vi "클라우드_날씨예보서비스.vi"() -> ()   [LabVIEW 2023]
uses:
  <vilib>/xml/Load XML String.vi
  <vilib>/xml/Close Reference(Node).vi
  System.Windows.Forms
  <vilib>/httpClient/LabVIEWHTTPClient.lvlib
  <vilib>/ni/Simple XML/Simple XML.lvlib
  <vilib>/xml/NI_XML.lvlib
  <resource>/objmgr/DOMUserDefRef.rc
panel:
  in  "격자 Y":string
  in  "격자 X":string
  out "초단기예보":T1(array[cluster])
  out "array":cluster{"이름":string, "node text":string}[][](array[cluster])
  out "Pretty XML String":string
  out "body":string
  out "header":string
  in  "경도":string
  in  "위도":string
  in  "새로고침":bool
  in  "정지 버튼":bool
  in  "웹 브라우저":refnum<k24>(container)
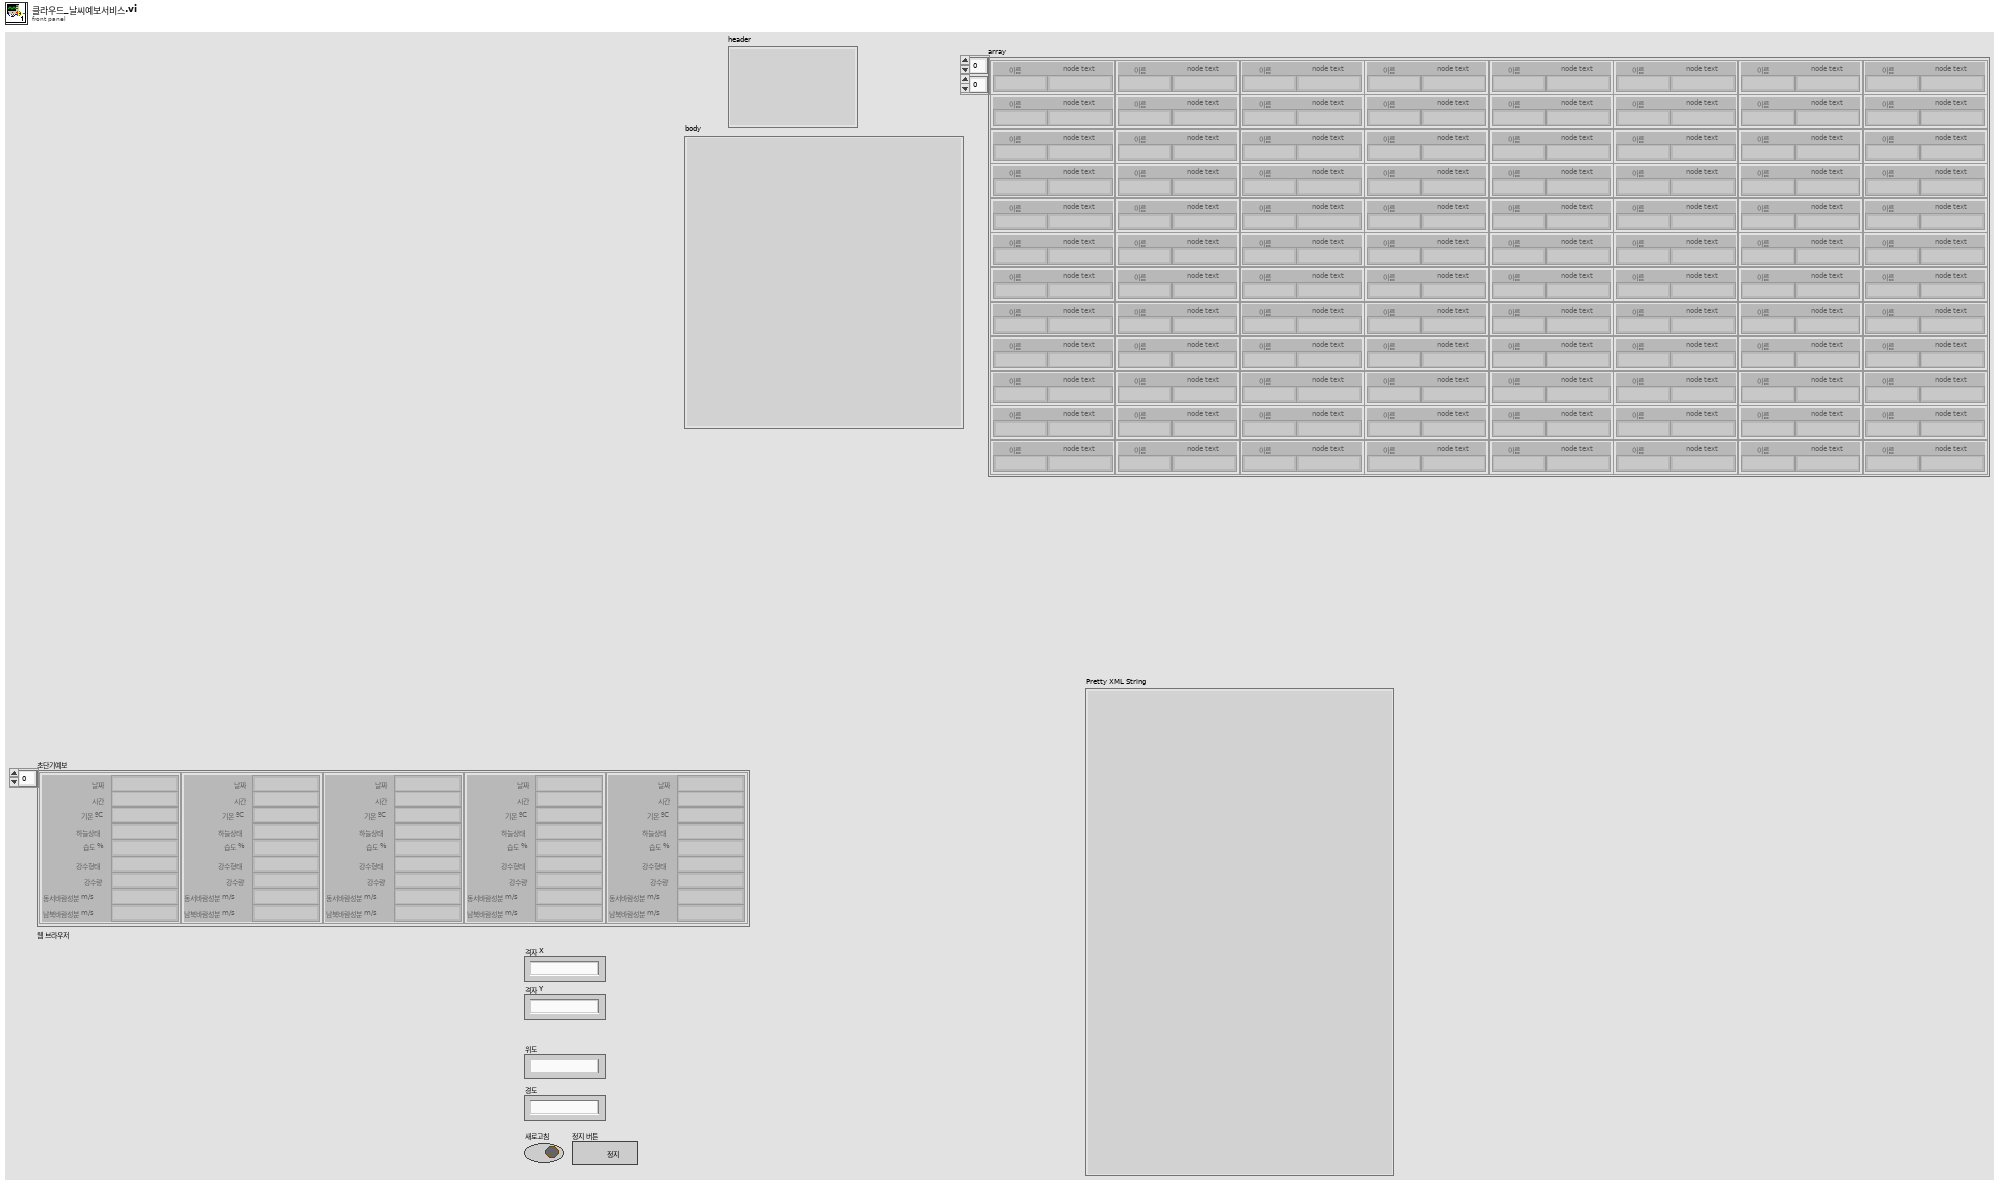
[diagram p1: front panel]
types:
  T1 = cluster{"날짜":string, "시간":string, "기온 ºC":string, "하늘상태":string, "습도 %":string, "강수형태":string, "강수량":string, "동서바람성분 m/s":string, "남북바람성분 m/s":string}[]
  T2 = cluster{"node text":string, "node text":string, "node text":string, string, "node text":string, string, string, "node text":string, "node text":string}
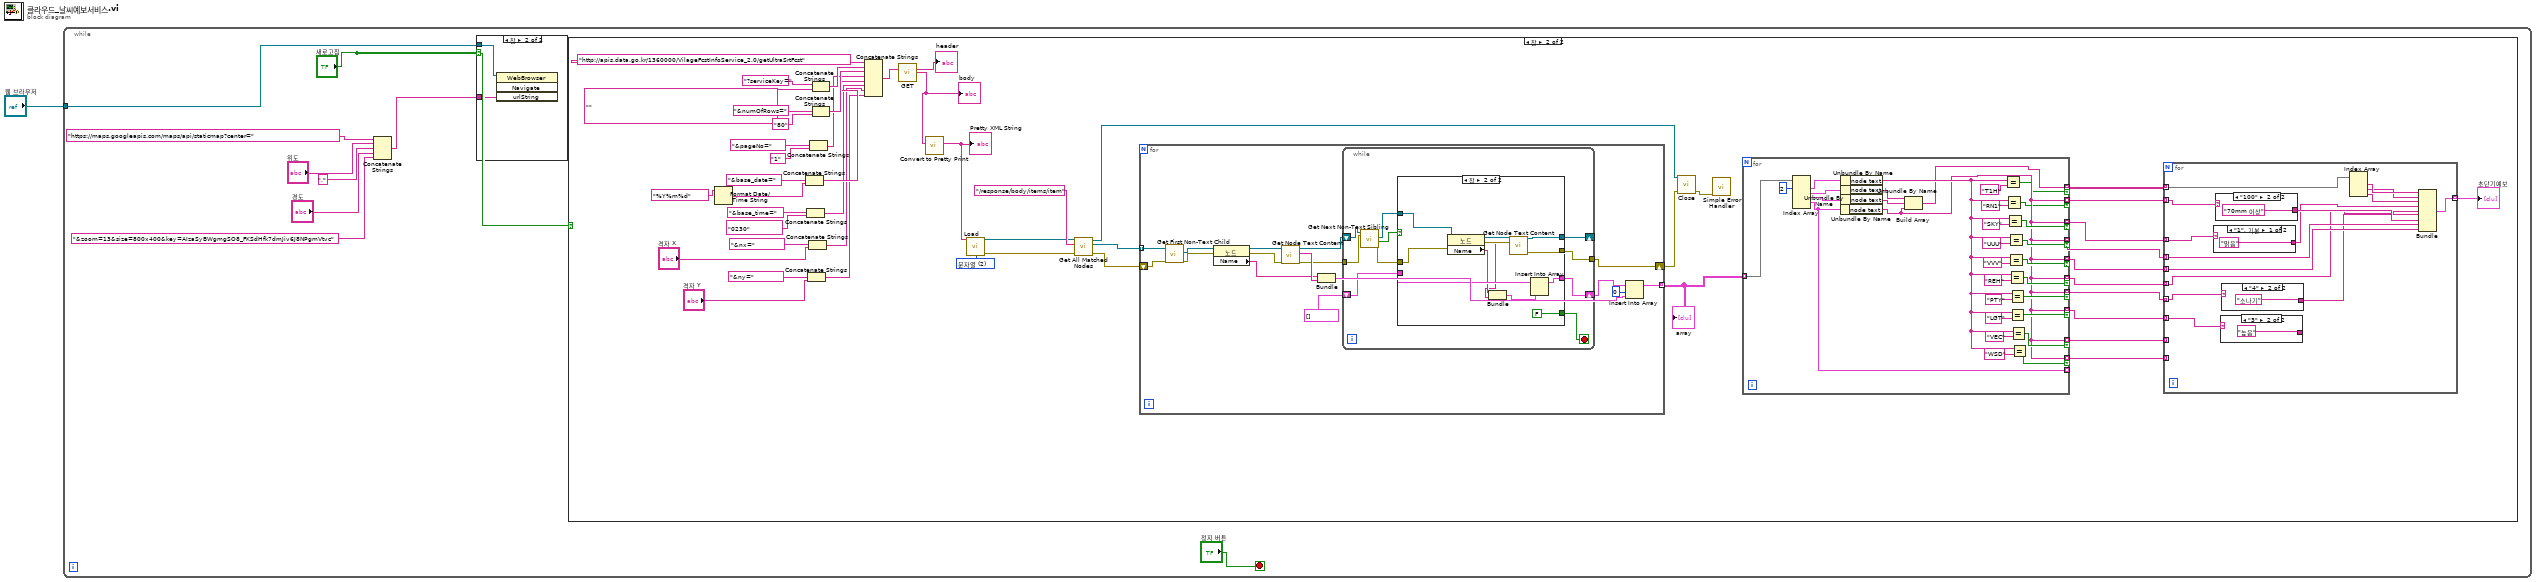
[diagram p0: block diagram]
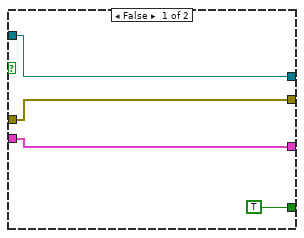
[diagram p7: hidden frame]
diagram:
  n1 = while {
    tunnel: "웹 브라우저" -> [w4]
    stop <- "정지 버튼" stop-if-true
    n2 = Concatenate Strings("https://maps.googleapis.com/maps/api/staticmap?center=", "위도", ",", "경도", "&zoom=13&size=800x400&key=AIzaSyBWgmgSO8_FKSdHfk7dmJiv6J8NPgmVtvc") -> (w3:string)
    n3 = case shown="참" "새로고침" {
      tunnel: w4 -> [_ w156]
      tunnel: w3 -> [_ w155]
      frame False {
      }
      frame True {
        n4 = invoke class="WebBrowser" method="Navigate"(reference=w156, "urlString"=w155) -> ()  [unwired: 2 in, 4 out]
      }
    }
    n5 = case shown="참" "새로고침" {
      frame False {
      }
      frame True {
        w46 = 2 items=["Never", "Always", "문자열"] ("validate on load (Auto)")
        n6 = Format Date/Time String(time format string (%c)="%Y%m%d") -> (date/time string=w11:string)  [unwired: 2 in]
        n7 = Concatenate Strings("&base_date=", w11) -> (w31:string)
        n8 = Concatenate Strings("&base_time=", "0230") -> (w30:string)
        n9 = Concatenate Strings("&ny=", "격자 Y") -> (w28:string)
        n10 = Concatenate Strings("&nx=", "격자 X") -> (w29:string)
        n11 = Concatenate Strings("&pageNo=", "1") -> (w32:string)
        n12 = Concatenate Strings("?serviceKey=", "") -> (w55:string)
        n13 = Concatenate Strings("&numOfRows=", "80") -> (w56:string)
        n14 = Concatenate Strings("http://apis.data.go.kr/1360000/VilageFcstInfoService_2.0/getUltraSrtFcst", w55, w56, w32, w31, w30, w29, w28) -> (w58:string)
        n15 = call <vilib>:"GET.vi"("url"=w58) -> ("headers"=→"header":string, "body"=w27:string)  [unwired: 11 in, 2 out]
        "body" <- w27
        n16 = call <vilib>:"Convert to Pretty Print.vi"("XML String"=w27) -> ("Pretty XML String"=w45:string)  [unwired: 9 in, 1 out]
        "Pretty XML String" <- w45
        n17 = call-poly <vilib>:"Load.vi"("XML string"=w45, "validate on load (Auto)"=w46) -> ("DOM document out"=w48:refnum<k20>, "error out"=w47:errorcluster)  [unwired: 11 in, 1 out]
        n18 = call <vilib>:"Get All Matched Nodes.vi"("error in (no error)"=w47, "XPath expression"="/response/body/items/item", "node in"=w48) -> ("error out"=w44:errorcluster, "node result array"=w43:refnum<k20>[], "node out"=w42:refnum<k20>)  [unwired: 6 in]
        n19 = for {
          tunnel: w43 -> [w128] mode=indexing
          shift-right: [w114] -> w40
          shift-left: w44 -> [w127]
          tunnel: [w113] -> w26 mode=indexing
          n20 = call <vilib>:"Get First Non-Text Child.vi"("error in (no error)"=w127, "node in"=w128) -> ("error out"=w126:errorcluster, "child node"=w125:refnum<k20>)  [unwired: 6 in, 2 out]
          n21 = property class="노드"(reference=w125, error in=w126) -> (reference out=w124:refnum<k20>, error out=w123:errorcluster, "Name"=w121:string)
          n22 = call <vilib>:"Get Node Text Content.vi"("error in (no error)"=w123, "node in"=w124) -> ("error out"=w117:errorcluster, "node text"=w122:string, "node out"=w118:refnum<k20>)  [unwired: 7 in]
          n23 = Bundle("이름"=w121, "node text"=w122) -> (w119:cluster{"이름":string, "node text":string})  [unwired: 1 in]
          n24 = while {
            shift-right: [w132] -> _
            shift-left: w118 -> [w136]
            tunnel: w117 -> [w131]
            shift-right: [w134] -> w115
            shift-left: cluster{"Name":string, "node text":string}[] [] ("array") -> [w137]
            tunnel: [w133] -> w114
            stop <- w138 stop-if-true
            n25 = call <vilib>:"Get Next Non-Text Sibling.vi"("error in (no error)"=w131, "node in"=w136) -> ("error out"=w130:errorcluster, "found sibling node?"=w129:bool, "sibling node"=w135:refnum<k20>)  [unwired: 6 in, 1 out]
            n26 = case shown="참" w129 {
              tunnel: [TRUE FALSE] -> w138
              tunnel: w137 -> [w141 w151]
              tunnel: w130 -> [w140 w153]
              tunnel: w135 -> [w139 w152]
              tunnel: [w140 w146] -> w133
              tunnel: [w141 w144] -> w134
              tunnel: [w139 w143] -> w132
              frame False {
              }
              frame True {
                n27 = property class="노드"(reference=w152, error in=w153) -> (reference out=w149:refnum<k20>, error out=w150:errorcluster, "Name"=w148:string)
                n28 = call <vilib>:"Get Node Text Content.vi"("error in (no error)"=w150, "node in"=w149) -> ("error out"=w146:errorcluster, "node text"=w147:string, "node out"=w143:refnum<k20>)  [unwired: 7 in]
                n29 = Bundle("이름"=w148, "node text"=w147) -> (w145:cluster{"이름":string, "node text":string})  [unwired: 1 in]
                n30 = Insert Into Array(array=w151, new element=w145) -> (w144:cluster{"Name":string, "node text":string}[])  [unwired: 1 in]
              }
            }
          }
          n31 = Insert Into Array(array=w115, index=0, new element=w119) -> (w113:cluster{"Name":string, "node text":string}[])
        }
        "array" <- w26
        n32 = call-poly <vilib>:"Close.vi"("error in (no error)"=w40, "node"=w42) -> ("error out"=w41:errorcluster)  [unwired: 7 in]
        n33 = call <vilib>:"Simple Error Handler.vi"("error in (no error)"=w41) -> ()  [unwired: 4 in, 5 out]
        n34 = for {
          tunnel: w26 -> [w112] mode=indexing
          tunnel: [w85] -> w25 mode=indexing if=w83
          tunnel: [w86] -> w24 mode=indexing if=w82
          tunnel: [w86] -> w23 mode=indexing if=w94
          tunnel: [w86] -> w22 mode=indexing if=w93
          tunnel: [w86] -> w21 mode=indexing if=w92
          tunnel: [w86] -> w20 mode=indexing if=w91
          tunnel: [w86] -> w19 mode=indexing if=w90
          tunnel: [w86] -> w18 mode=indexing if=w89
          tunnel: [w86] -> w17 mode=indexing if=w88
          tunnel: [w86] -> w16 mode=indexing if=w87
          tunnel: [w84] -> _ mode=indexing
          n35 = Index Array(array=w112, index #1=2 ("index")) -> (element #1=w110:cluster{"Name":string, "node text":string}, element #2=w109:cluster{"Name":string, "node text":string}, element #3=w108:cluster{"Name":string, "node text":string}, element #4=w84:cluster{"Name":string, "node text":string})  [unwired: 4 in, 1 out]
          n36 = Unbundle By Name(w84) -> ("node text"=w86:string)
          n37 = Unbundle By Name(w110) -> ("node text"=w96:string)
          n38 = Unbundle By Name(w109) -> ("node text"=w107:string)
          n39 = Unbundle By Name(w108) -> ("node text"=w106:string)
          n40 = Build Array(w107, w106, w86) -> (w85:string[])
          n41 = Equal?(x=w96, y="T1H") -> (x = y?=w83:bool)
          n42 = Equal?(x=w96, y="RN1") -> (x = y?=w82:bool)
          n43 = Equal?(x=w96, y="SKY") -> (x = y?=w94:bool)
          n44 = Equal?(x=w96, y="UUU") -> (x = y?=w93:bool)
          n45 = Equal?(x=w96, y="VVV") -> (x = y?=w92:bool)
          n46 = Equal?(x=w96, y="REH") -> (x = y?=w91:bool)
          n47 = Equal?(x=w96, y="PTY") -> (x = y?=w90:bool)
          n48 = Equal?(x=w96, y="LGT") -> (x = y?=w89:bool)
          n49 = Equal?(x=w96, y="VEC") -> (x = y?=w88:bool)
          n50 = Equal?(x=w96, y="WSD") -> (x = y?=w87:bool)
        }
        n51 = for {
          tunnel: w25 -> [w73] mode=indexing
          tunnel: [w72] -> w15 mode=indexing
          tunnel: w24 -> [w71] mode=indexing
          tunnel: w23 -> [w70] mode=indexing
          tunnel: w22 -> [w66] mode=indexing
          tunnel: w21 -> [w67] mode=indexing
          tunnel: w20 -> [w63] mode=indexing
          tunnel: w19 -> [w68] mode=indexing
          tunnel: w18 -> [w69] mode=indexing
          tunnel: w17 -> [_] mode=indexing
          tunnel: w16 -> [_] mode=indexing
          n52 = case shown="\"1\", 기본" w70 {
            selector: w70 -> [_ w79]
            tunnel: ["맑음" w79] -> w62
            frame "1", Default {
            }
            frame "100" {
            }
          }
          n53 = case shown="\"100\"" w71 {
            selector: w71 -> [w80 _]
            tunnel: [w80 "70mm 이상"] -> w65
            frame "False", Default {
            }
            frame "100" {
            }
          }
          n54 = case shown="\"3\"" w69 {
            selector: w69 -> [w74 _]
            tunnel: [w74 "높음"] -> _
            frame "1", Default {
            }
            frame "3" {
            }
          }
          n55 = case shown="\"4\"" w68 {
            selector: w68 -> [w76 _]
            tunnel: [w76 "소나기"] -> w64
            frame "1", Default {
            }
            frame "4" {
            }
          }
          n56 = Index Array(array=w73) -> (element #1=w61:string, element #2=w60:string, element #3=w59:string)  [unwired: 3 in]
          n57 = Bundle("node text"=w61, "node text"=w60, "node text"=w59, w62, "node text"=w63, w64, w65, "node text"=w66, "node text"=w67) -> (w72:T2)  [unwired: 1 in]
        }
        "초단기예보" <- w15
      }
    }
  }
